vi "Sort Updated Time Descending.vi"(10 "Panel B":refnum<class "Panel.lvclass">, 11 "Panel A":refnum<class "Panel.lvclass">) -> (3 "A < B":bool)   [LabVIEW 2020, in "PicoG-Processor.lvlib"]
uses:
  PicoG-Processor.lvlib
  <vilib>/IlluminatedG/IG OOPanel/OOPanel/Panel/Panel.lvclass
  WebProjectPanel/WebProjectPanel.lvclass
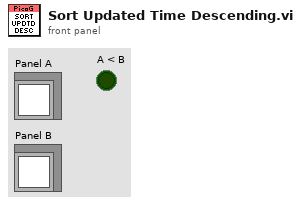
[diagram p1: front panel]
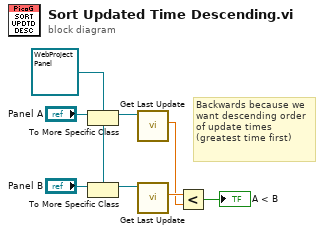
[diagram p0: block diagram]
diagram:
  w6 = refnum<class "WebProjectPanel.lvclass"> refnum ("PicoG-Processor:WebProjectPanel")
  # "Backwards because we want descending order of update times (greatest time first)"
  n1 = To More Specific Class(target class=w6, reference="Panel A") -> (specific class reference=w5:refnum<class "WebProjectPanel.lvclass">)  [unwired: 1 in, 1 out]
  n2 = To More Specific Class(target class=w6, reference="Panel B") -> (specific class reference=w4:refnum<class "WebProjectPanel.lvclass">)  [unwired: 1 in, 1 out]
  n3 = call "Get Last Update.vi"("WebProjectPanel in"=w5) -> ("Last Update"=w2:dbl)  [unwired: 8 in, 2 out]
  n4 = call "Get Last Update.vi"("WebProjectPanel in"=w4) -> ("Last Update"=w3:dbl)  [unwired: 8 in, 2 out]
  n5 = Less?(x=w3, y=w2) -> (x < y?=→"A < B":bool)
